vi "Set Value.vi"(8 "error in":errorcluster, 10 "Value":variant, 11 "Check Box in":refnum<class "Check Box.lvclass">) -> (0 "error out":errorcluster, 3 "Check Box out":refnum<class "Check Box.lvclass">)   [LabVIEW 2024, in "SourceGrid.lvlib" / "Check Box.lvclass"]
uses:
  Check Box.lvclass
  D:/git/Sourcegrid-LabVIEW/dll/SourceGrid.dll
  dll/SourceGrid.dll
  Check Box.lvclass/Check Box.ctl
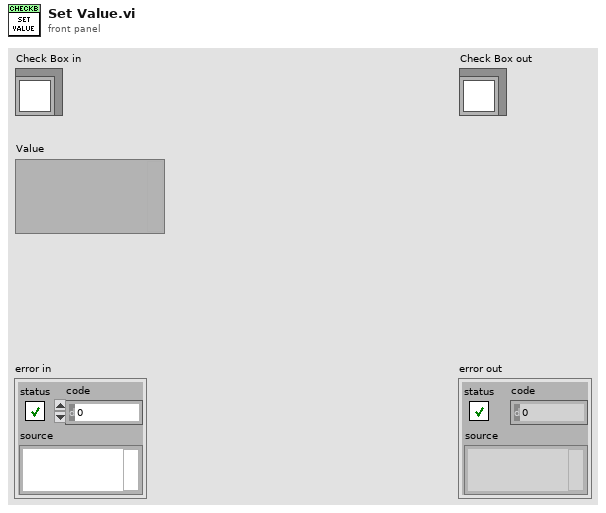
[diagram p1: front panel]
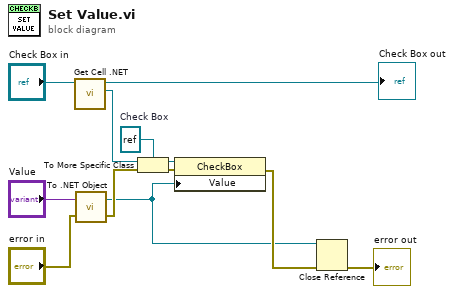
[diagram p0: block diagram]
diagram:
  w6 = refnum<k24> refnum  # Check Box
  n1 = call-dynamic "Get Cell .NET.vi"("Cell in"="Check Box in") -> ("Cell .NET"=w9:refnum<k24>, "Cell out"=→"Check Box out":refnum<class "Check Box.lvclass">)  [unwired: 9 in]
  n2 = call <vilib>:"To .NET Object.vi"("error in (no error)"="error in", "anything"="Value") -> ("error out"=w5:errorcluster, ".NET object"=w1:refnum<k24>)
  n3 = To More Specific Class(target class=w6, reference=w9, error in=w5) -> (specific class reference=w7:refnum<k24>, error out=w4:errorcluster)
  n4 = property class="CheckBox"(reference=w7, error in=w4, "Value"=w1) -> (error out=w3:errorcluster)  [unwired: 1 out]
  n5 = Close Reference(reference=w1, error in (no error)=w3) -> (error out=→"error out":errorcluster)
